vi "File_BuildNewPath.vi"(1 "Path":path, 2 "Top Source Folder":path, 3 "Top Target Folder":path, 4 "Include Top Source Folder?":bool=TRUE) -> (15 "New path":path)   [LabVIEW 2014]
doc: "Builds a new path by replaceing the Top source path with new top target path."
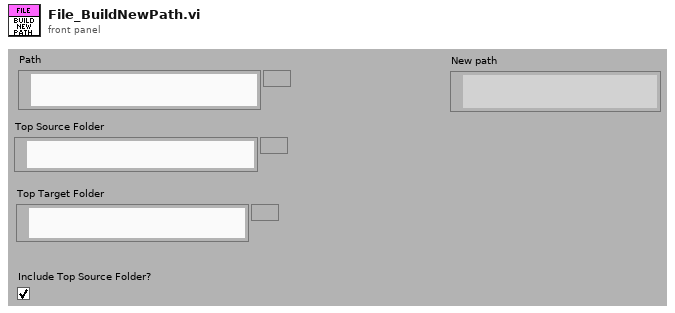
[diagram p1: front panel]
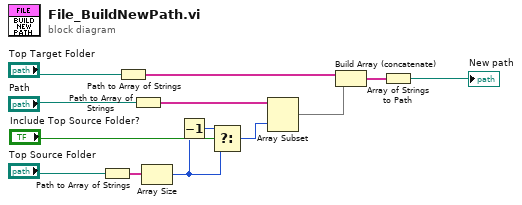
[diagram p0: block diagram]
diagram:
  n1 = Path to Array of Strings(0:"Top Source Folder") -> (2:w10:string[])  [unwired: 1 out]
  n2 = Path to Array of Strings(0:"Top Target Folder") -> (2:w8:string[])  [unwired: 1 out]
  n3 = Path to Array of Strings(0:"Path") -> (2:w9:string[])  [unwired: 1 out]
  n4 = Array Size(array=w10) -> (size(s)=w2:i32)
  n5 = Decrement(x=w2) -> (x-1=w3:i32)
  n6 = Select(t=w3, s="Include Top Source Folder?", f=w2) -> (s? t:f=w1:i32)
  n7 = Array Subset(array=w9, index=w1) -> (w7:string[])  [unwired: 1 in]
  n8 = Build Array (concatenate)(w8, w7) -> (w6:string[])
  n9 = Array of Strings to Path(0:w6) -> (2:→"New path":path)  [unwired: 1 in]
